vi "gameLoop.vi"() -> ()   [LabVIEW 2015]
uses:
  colorbox cluster.ctl
panel:
  out "2048 2":T1[][](array[typedef])
  in  "Stop Button":bool
  out "2048":dbl[][](array[numeric])
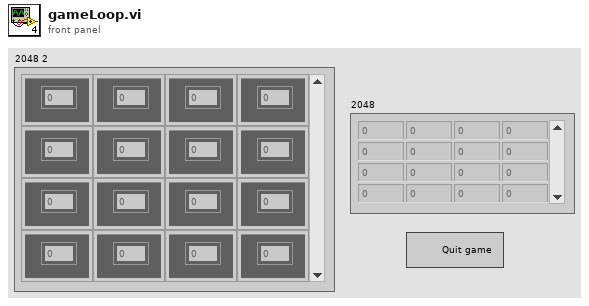
[diagram p1: front panel]
types:
  T1 = typedef "colorbox cluster.ctl" = cluster{"Color Box":u32, "Numeric":dbl}
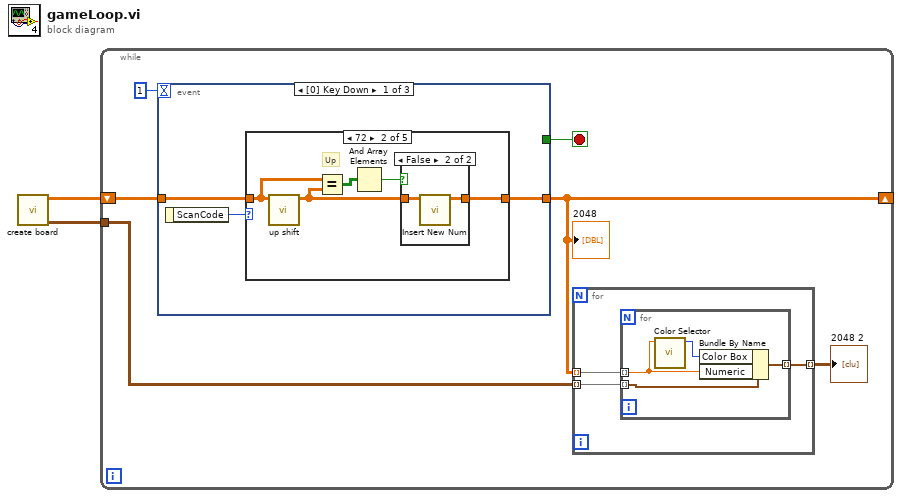
[diagram p0: block diagram]
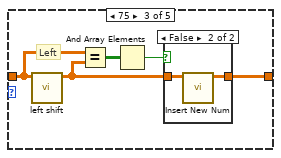
[diagram p4: hidden frame]
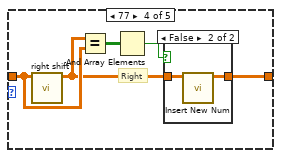
[diagram p6: hidden frame]
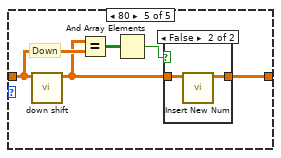
[diagram p8: hidden frame]
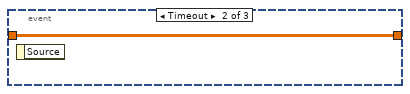
[diagram p10: hidden frame]
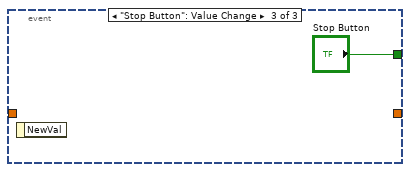
[diagram p11: hidden frame]
diagram:
  n1 = call "create board.vi"() -> ("2048 2"=w1:T1[][], "board"=w2:dbl[][])  [unwired: 10 in]
  n2 = while {
    shift-right: [w4] -> _
    shift-left: w2 -> [w7]
    tunnel: w1 -> [w5]
    stop <- w8 stop-if-true
    n3 = event shown="[0] Key Down" {
      selector: _ -> [_ _ _]
      dyn-events: _ -> [_ _ _]
      timeout: 1 -> [_ _ _]
      tunnel: [_ _ "Stop Button"] -> w8
      tunnel: w7 -> [w17 w52 _]
      tunnel: [w16 w52 _] -> w4
      event Key Down {
        n4 = event-data() -> ("ScanCode"=w18:i16)  [unwired: 1 in]
        n5 = case shown="72" w18 {
          tunnel: w17 -> [w19 w23 w31 w39 w47]
          tunnel: [w19 w24 w32 w40 w48] -> w16
          frame 0, Default {
          }
          frame 72 {
            # "Up"
            n6 = call "up shift.vi"("2048 2"=w23) -> ("2048"=w20:dbl[][])  [unwired: 10 in]
            n7 = Equal?(x=w23, y=w20) -> (x = y?=w21:bool[][])
            n8 = And Array Elements(Boolean array=w21) -> (logical AND=w22:bool)
            n9 = case shown="False" w22 {
              tunnel: [w25 w27] -> w24
              tunnel: w20 -> [w25 w26]
              frame True {
              }
              frame False {
                n10 = call "Insert New Num.vi"("board in"=w26) -> ("board out"=w27:dbl[][])  [unwired: 10 in]
              }
            }
          }
          frame 75 {
            # "Left"
            n11 = call "left shift.vi"("2048 2"=w31) -> ("2048"=w28:dbl[][])  [unwired: 10 in]
            n12 = Equal?(x=w31, y=w28) -> (x = y?=w30:bool[][])
            n13 = And Array Elements(Boolean array=w30) -> (logical AND=w29:bool)
            n14 = case shown="False" w29 {
              tunnel: [w33 w35] -> w32
              tunnel: w28 -> [w33 w34]
              frame True {
              }
              frame False {
                n15 = call "Insert New Num.vi"("board in"=w34) -> ("board out"=w35:dbl[][])  [unwired: 10 in]
              }
            }
          }
          frame 77 {
            # "Right"
            n16 = call "right shift.vi"("2048 2"=w39) -> ("2048"=w36:dbl[][])  [unwired: 10 in]
            n17 = Equal?(x=w36, y=w39) -> (x = y?=w38:bool[][])
            n18 = And Array Elements(Boolean array=w38) -> (logical AND=w37:bool)
            n19 = case shown="False" w37 {
              tunnel: [w41 w43] -> w40
              tunnel: w36 -> [w41 w42]
              frame True {
              }
              frame False {
                n20 = call "Insert New Num.vi"("board in"=w42) -> ("board out"=w43:dbl[][])  [unwired: 10 in]
              }
            }
          }
          frame 80 {
            # "Down"
            n21 = call "down shift.vi"("2048 2"=w47) -> ("2048"=w44:dbl[][])  [unwired: 10 in]
            n22 = Equal?(x=w44, y=w47) -> (x = y?=w46:bool[][])
            n23 = And Array Elements(Boolean array=w46) -> (logical AND=w45:bool)
            n24 = case shown="False" w45 {
              tunnel: [w49 w51] -> w48
              tunnel: w44 -> [w49 w50]
              frame True {
              }
              frame False {
                n25 = call "Insert New Num.vi"("board in"=w50) -> ("board out"=w51:dbl[][])  [unwired: 10 in]
              }
            }
          }
        }
      }
      event Timeout {
        n26 = event-data() -> ()  [unwired: 1 in, 1 out]
      }
      event "Stop Button": Value Change {
        n27 = event-data() -> ()  [unwired: 1 in, 1 out]
      }
    }
    "2048" <- w4
    n28 = for {
      tunnel: w5 -> [w11] mode=indexing
      tunnel: w4 -> [w10] mode=indexing
      tunnel: [w9] -> w3 mode=indexing
      n29 = for {
        tunnel: w11 -> [w15] mode=indexing
        tunnel: w10 -> [w12] mode=indexing
        tunnel: [w14] -> w9 mode=indexing
        n30 = call "Color Selector.vi"("Numeric Control"=w12) -> ("Color Box"=w13:u32)  [unwired: 10 in]
        n31 = Bundle By Name(cluster=w15, "Color Box"=w13, "Numeric"=w12) -> (w14:T1)
      }
    }
    "2048 2" <- w3
  }
